vi "CTRE_CAN_GetThreeParam20.vi"(8 "error in (no error)":errorcluster, 11 "ArbID":u32 format="%.0x") -> (0 "error out":errorcluster, 2 "3Params":i32[](array[numeric]), 3 "ArbID Out":u32 format="%.0x")   [LabVIEW 2016]
panel:
  out "Param 3":u32
  out "Param 2":u32
  out "Param1":u32
  out "3Params_":u32[](array[numeric])
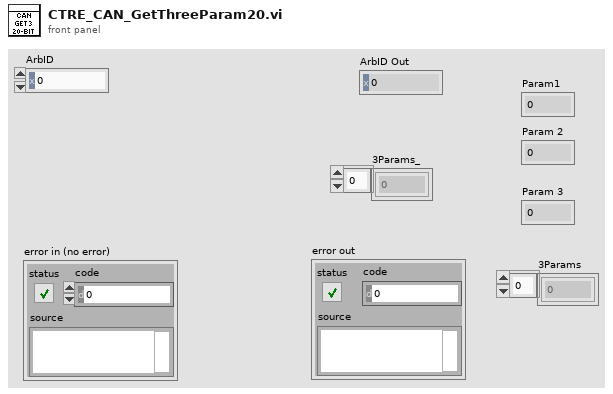
[diagram p1: front panel]
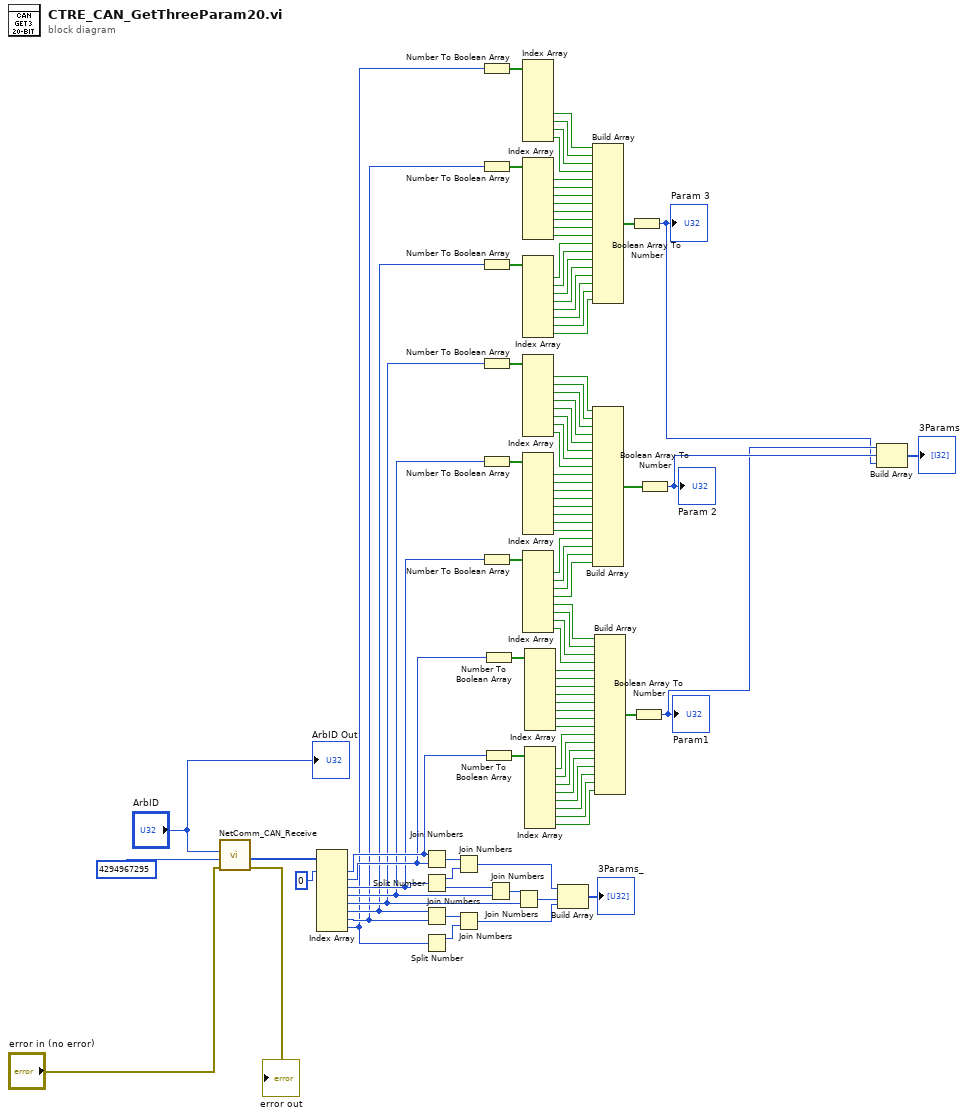
[diagram p0: block diagram]
diagram:
  n1 = call <vilib>:"NetComm_CAN_Receive.vi"("error in (no error)"="error in (no error)", "Message ID Mask"=u32 4294967295, "Message ID"="ArbID") -> ("error out"=→"error out":errorcluster, "Data"=w95:u8[])  [unwired: 5 in, 2 out]
  n2 = Index Array(array=w95, index #1=0 ("index")) -> (element #1=w82:u8, element #2=w80:u8, element #3=w79:u8, element #4=w54:u8, element #5=w53:u8, element #6=w28:u8, element #7=w27:u8, element #8=w26:u8)  [unwired: 7 in]
  n3 = Join Numbers(hi=w82, lo=w80) -> ((hi.lo)=w97:u16)
  n4 = Split Number(x=w79) -> (hi(x)=w92:u8, lo(x)=w91:u8)
  n5 = Join Numbers(hi=w28, lo=w27) -> ((hi.lo)=w99:u16)
  n6 = Split Number(x=w26) -> (hi(x)=w90:u8)  [unwired: 1 out]
  n7 = Join Numbers(hi=w97, lo=w92) -> ((hi.lo)=w86:u32)
  n8 = Join Numbers(hi=w99, lo=w90) -> ((hi.lo)=w85:u32)
  n9 = Number To Boolean Array(number=w26) -> (Boolean array=w31:bool[])
  n10 = Number To Boolean Array(number=w27) -> (Boolean array=w30:bool[])
  n11 = Number To Boolean Array(number=w28) -> (Boolean array=w29:bool[])
  n12 = Number To Boolean Array(number=w53) -> (Boolean array=w55:bool[])
  n13 = Number To Boolean Array(number=w54) -> (Boolean array=w56:bool[])
  n14 = Number To Boolean Array(number=w79) -> (Boolean array=w78:bool[])
  n15 = Number To Boolean Array(number=w80) -> (Boolean array=w81:bool[])
  n16 = Number To Boolean Array(number=w82) -> (Boolean array=w83:bool[])
  n17 = Join Numbers(hi=w91, lo=w54) -> ((hi.lo)=w98:u16)
  n18 = Join Numbers(hi=w98, lo=w53) -> ((hi.lo)=w87:u32)
  n19 = Index Array(array=w31) -> (element #5=w5:bool, element #6=w6:bool, element #7=w7:bool, element #8=w8:bool)  [unwired: 8 in, 4 out]
  n20 = Index Array(array=w30) -> (element #1=w9:bool, element #2=w10:bool, element #3=w11:bool, element #4=w12:bool, element #5=w13:bool, element #6=w14:bool, element #7=w15:bool, element #8=w16:bool)  [unwired: 8 in]
  n21 = Index Array(array=w29) -> (element #1=w17:bool, element #2=w18:bool, element #3=w19:bool, element #4=w20:bool, element #5=w21:bool, element #6=w22:bool, element #7=w23:bool, element #8=w24:bool)  [unwired: 8 in]
  n22 = Index Array(array=w55) -> (element #1=w33:bool, element #2=w34:bool, element #3=w35:bool, element #4=w36:bool, element #5=w37:bool, element #6=w38:bool, element #7=w39:bool, element #8=w40:bool)  [unwired: 8 in]
  n23 = Index Array(array=w56) -> (element #1=w41:bool, element #2=w42:bool, element #3=w43:bool, element #4=w44:bool, element #5=w45:bool, element #6=w46:bool, element #7=w47:bool, element #8=w48:bool)  [unwired: 8 in]
  n24 = Index Array(array=w78) -> (element #1=w49:bool, element #2=w50:bool, element #3=w51:bool, element #4=w52:bool, element #5=w57:bool, element #6=w58:bool, element #7=w59:bool, element #8=w60:bool)  [unwired: 8 in]
  n25 = Index Array(array=w81) -> (element #1=w61:bool, element #2=w62:bool, element #3=w63:bool, element #4=w64:bool, element #5=w65:bool, element #6=w66:bool, element #7=w67:bool, element #8=w68:bool)  [unwired: 8 in]
  n26 = Index Array(array=w83) -> (element #1=w69:bool, element #2=w70:bool, element #3=w71:bool, element #4=w72:bool, element #5=w73:bool, element #6=w74:bool, element #7=w75:bool, element #8=w76:bool)  [unwired: 8 in]
  n27 = Build Array(w86, w87, w85) -> (→"3Params_":u32[])
  n28 = Build Array(w5, w6, w7, w8, w9, w10, w11, w12, w13, w14, w15, w16, w17, w18, w19, w20, w21, w22, w23, w24) -> (w25:bool[])
  n29 = Build Array(w33, w34, w35, w36, w37, w38, w39, w40, w41, w42, w43, w44, w45, w46, w47, w48, w49, w50, w51, w52) -> (w32:bool[])
  n30 = Build Array(w57, w58, w59, w60, w61, w62, w63, w64, w65, w66, w67, w68, w69, w70, w71, w72, w73, w74, w75, w76) -> (w77:bool[])
  n31 = Boolean Array To Number(Boolean array=w25) -> (number=w1:i32)
  "Param 3" <- w1
  n32 = Boolean Array To Number(Boolean array=w77) -> (number=w2:i32)
  "Param1" <- w2
  n33 = Boolean Array To Number(Boolean array=w32) -> (number=w3:i32)
  "Param 2" <- w3
  n34 = Build Array(w2, w3, w1) -> (→"3Params":i32[])
  "ArbID Out" <- "ArbID"
